vi "Send Remote Reply.vi"(7 "Original Payload":T1, 8 "error in (no error)":errorcluster, 9 "Message Type":string, 10 "Message":refnum<class "Message.lvclass">, 11 "Module in":refnum<class "Module.lvclass">) -> (0 "error out":errorcluster, 3 "Module out":refnum<class "Module.lvclass">)   [LabVIEW 2020, in "Volatus.lvlib" / "Module.lvclass"]
uses:
  Module.lvclass
  Module.lvclass/Module.ctl
  VolatusAPI/VolatusAPI.lvclass
  lv-vecto/Vecto/proto/TcpPayload/Data.ctl
  lv-vecto/Vecto/proto/TcpPayload/TcpPayload.lvlib
  lv-protoc/LV-Proto/Message/Message.lvclass
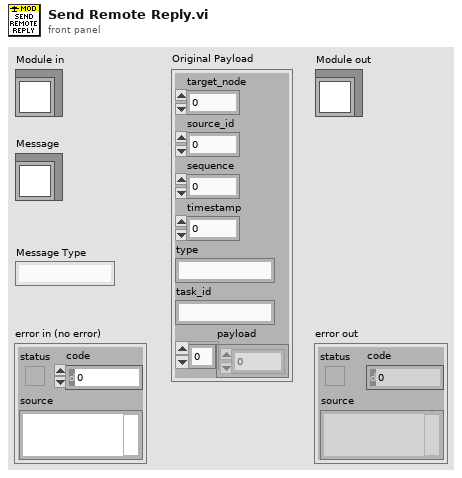
[diagram p1: front panel]
types:
  T1 = typedef "TcpPayload.lvlib/Data.ctl" = cluster{"target_node":u32, "source_id":u32, "sequence":u32, "timestamp":u64, "type":string, "task_id":string, "payload":u8[]}
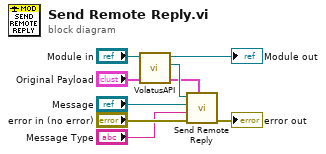
[diagram p0: block diagram]
diagram:
  n1 = call "VolatusAPI.vi"("Module in"="Module in") -> ("VolatusAPI"=w6:refnum<class "VolatusAPI.lvclass">, "Module out"=→"Module out":refnum<class "Module.lvclass">)  [unwired: 9 in]
  n2 = call "Send Remote Reply.vi"("Original Payload"="Original Payload", "error in (no error)"="error in (no error)", "Message Type"="Message Type", "Message"="Message", "VolatusAPI in"=w6) -> ("error out"=→"error out":errorcluster)  [unwired: 5 in, 1 out]
